vi "Vector Length.vi"(1 "Vector":cluster{"x":dbl, "y":dbl}={"x"=2.0, "y"=0.0}) -> (0 "||Vector||":dbl)   [LabVIEW 2009]
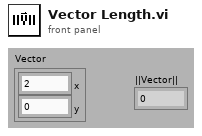
[diagram p1: front panel]
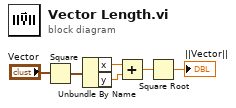
[diagram p0: block diagram]
diagram:
  n1 = Square(x="Vector") -> (x^2=w5:cluster{"x":dbl, "y":dbl})
  n2 = Unbundle By Name(w5) -> ("x"=w4:dbl, "y"=w3:dbl)
  n3 = Add(x=w4, y=w3) -> (x+y=w2:dbl)
  n4 = Square Root(x=w2) -> (sqrt(x)=→"||Vector||":dbl)
